vi "GetOverlay.vi"(8 "error in":errorcluster, 11 "NISE_CEF_Node in":refnum<class "NISE_CEF_Node.lvclass">) -> (0 "error out":errorcluster, 2 "overlay":string, 3 "NISE_CEF_Node out":refnum<class "NISE_CEF_Node.lvclass">)   [LabVIEW 2013, in "NISE_CEF_Node.lvclass"]
uses:
  NISE_CEF_Node.lvclass
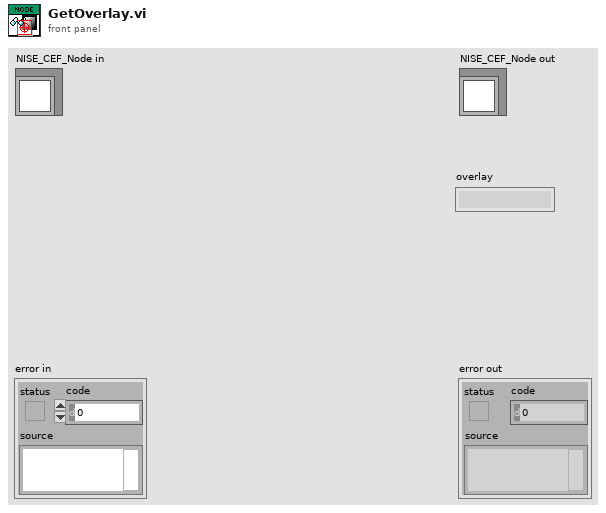
[diagram p1: front panel]
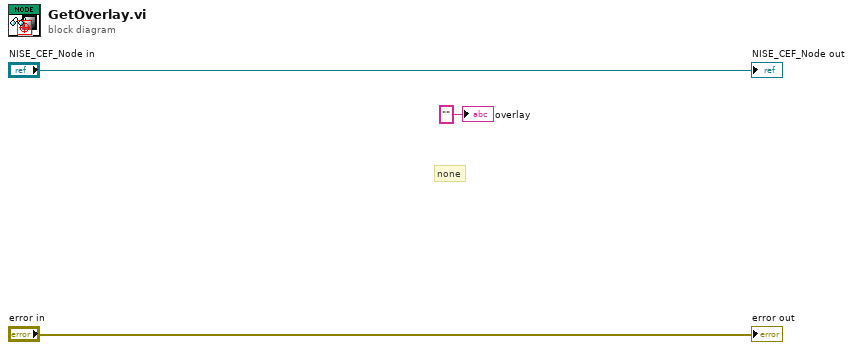
[diagram p0: block diagram]
diagram:
  # "none"
  "error out" <- "error in"
  "NISE_CEF_Node out" <- "NISE_CEF_Node in"
  "overlay" <- "" ("overlay")
